vi "Periodic Tasks.vi"(8 "error in":errorcluster) -> ()   [LabVIEW 2017]
doc: "This VI runs in parallel to other robot code. It can contain as many user-defined periodic loops as you need. These can carry out PID or other sorts of timed response."
uses:
  <vilib>/Rock Robotics/WPI/Utilities/WPI_GetSetVariantRefNum.vi
  <vilib>/Rock Robotics/Network Tables/NT Write Boolean.vi
  <vilib>/Rock Robotics/Network Tables/NT Write Number.vi
  <vilib>/Rock Robotics/Network Tables/NT Write String.vi
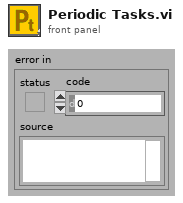
[diagram p1: front panel]
types:
  T1 = typedef "WPI_JoystickDevRef.ctl" = cluster{"Device":T2}
  T2 = typedef "WPI_JoystickDeviceEnum.ctl" = enum16{"USB 0", "USB 1", "USB 2", "USB 3", "USB 4", "USB 5"}
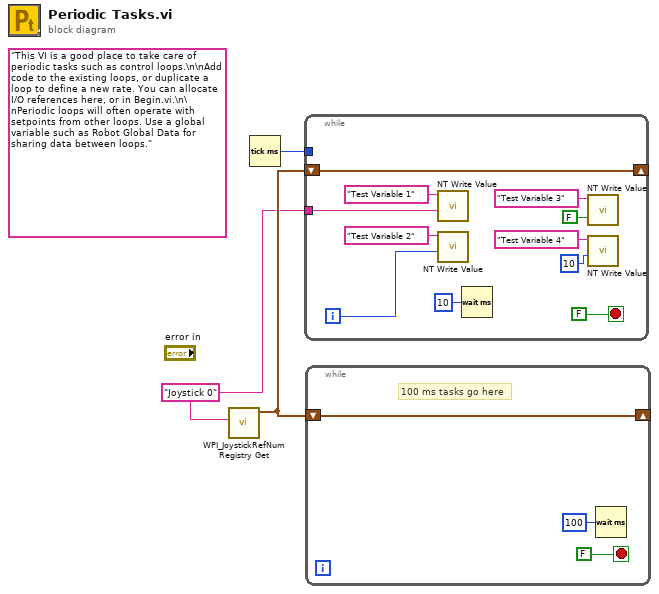
[diagram p0: block diagram]
diagram:
  (unwired) "This VI is a good place to take care of periodic tasks such as control loops.\n\nAdd code to the existing loops, or duplicate a loop to define a new rate. You can allocate I/O references here, or in Begin.vi.\n\nPeriodic loops will often operate with setpoints from other loops. Use a global variable such as Robot Global Data for sharing data between loops."
  w1 = "Joystick 0" ("refnum name")
  n1 = call <vilib>:"WPI_JoystickRefNum Registry Get.vi"("refnum name"=w1) -> ("JoystickDevRef"=w3:T1)  [unwired: 1 in, 9 out]
  n2 = Tick Count (ms)() -> (millisecond timer value=w2:u32)
  n3 = while {
    shift-right: [w13] -> _
    shift-left: w3 -> [w13]
    tunnel: w2 -> [_]
    tunnel: w1 -> [w8]
    i -> [w9]
    stop <- FALSE stop-if-true
    n4 = call-poly <vilib>:"NT Write Value.vi"("String"=w8, "Name"="Test Variable 1") -> ()  [unwired: 9 in, 1 out]
    n5 = call-poly <vilib>:"NT Write Value.vi"("Numeric"=w9, "Name"="Test Variable 2") -> ()  [unwired: 9 in, 1 out]
    n6 = Wait (ms)(milliseconds to wait=u32 10) -> ()  [unwired: 1 out]
    n7 = call-poly <vilib>:"NT Write Value.vi"("Boolean"=FALSE, "Name"="Test Variable 3") -> ()  [unwired: 9 in, 1 out]
    n8 = call-poly <vilib>:"NT Write Value.vi"("Numeric"=u32 10 ("milliseconds to wait"), "Name"="Test Variable 4") -> ()  [unwired: 9 in, 1 out]
  }
  n9 = while {
    shift-right: [w15] -> _
    shift-left: w3 -> [w15]
    stop <- FALSE stop-if-true
    # "100 ms tasks go here"
    n10 = Wait (ms)(milliseconds to wait=u32 100) -> ()  [unwired: 1 out]
  }
